vi "create_full_request_data.vi"(0 "llm_ollama_chatmodels in":refnum<class "llm_ollama_chatmodels.lvclass">, 5 "Messages":refnum<class "abstract_message_base.lvclass">[](array[class]), 11 "error in (no error)":errorcluster) -> (4 "llm_ollama_chatmodels out":refnum<class "llm_ollama_chatmodels.lvclass">, 6 "Request Data":string, 15 "error out":errorcluster)   [LabVIEW 2020, in "llm_ollama_chatmodels.lvclass"]
uses:
  llm_ollama_chatmodels.lvclass
  D:/Personal/LabVIEW LLMs/src/models/abstract_llm_base/abstract_llm_base.lvclass
  abstract_message_base/abstract_message_base.lvclass
  utils/ollama_chatmodel_request_data.ctl
  utils/ollama_options.ctl
  llm_ollama_chatmodels.lvclass/llm_ollama_chatmodels.ctl
  message_text/message_text.lvclass
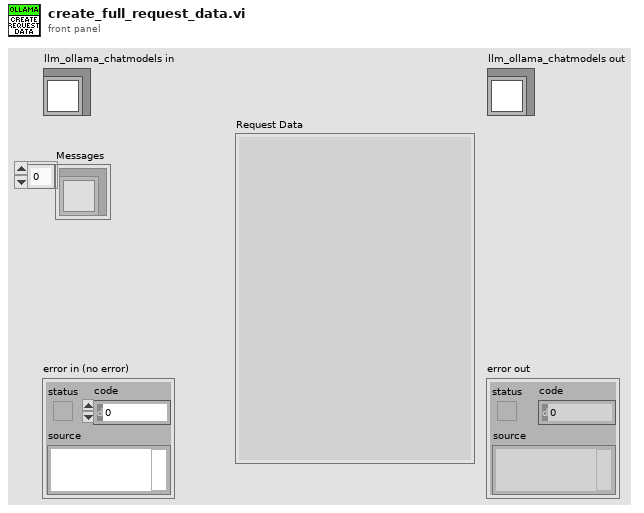
[diagram p1: front panel]
types:
  T1 = typedef "llm_ollama_chatmodels.lvclass/ollama_chatmodel_request_data.ctl" = cluster{"model":string, "messages":cluster{"role":string, "content":string}[], "stream":bool, "options":T2}
  T2 = typedef "llm_ollama_chatmodels.lvclass/ollama_options.ctl" = cluster{"temperature":dbl, "num_predict":i32, "top_p":dbl, "frequency_penalty":dbl, "presence_penalty":dbl, "seed":u32, "format":string}
  T3 = typedef "message_text.lvclass/message.ctl" = cluster{"role":string, "content":string[]}
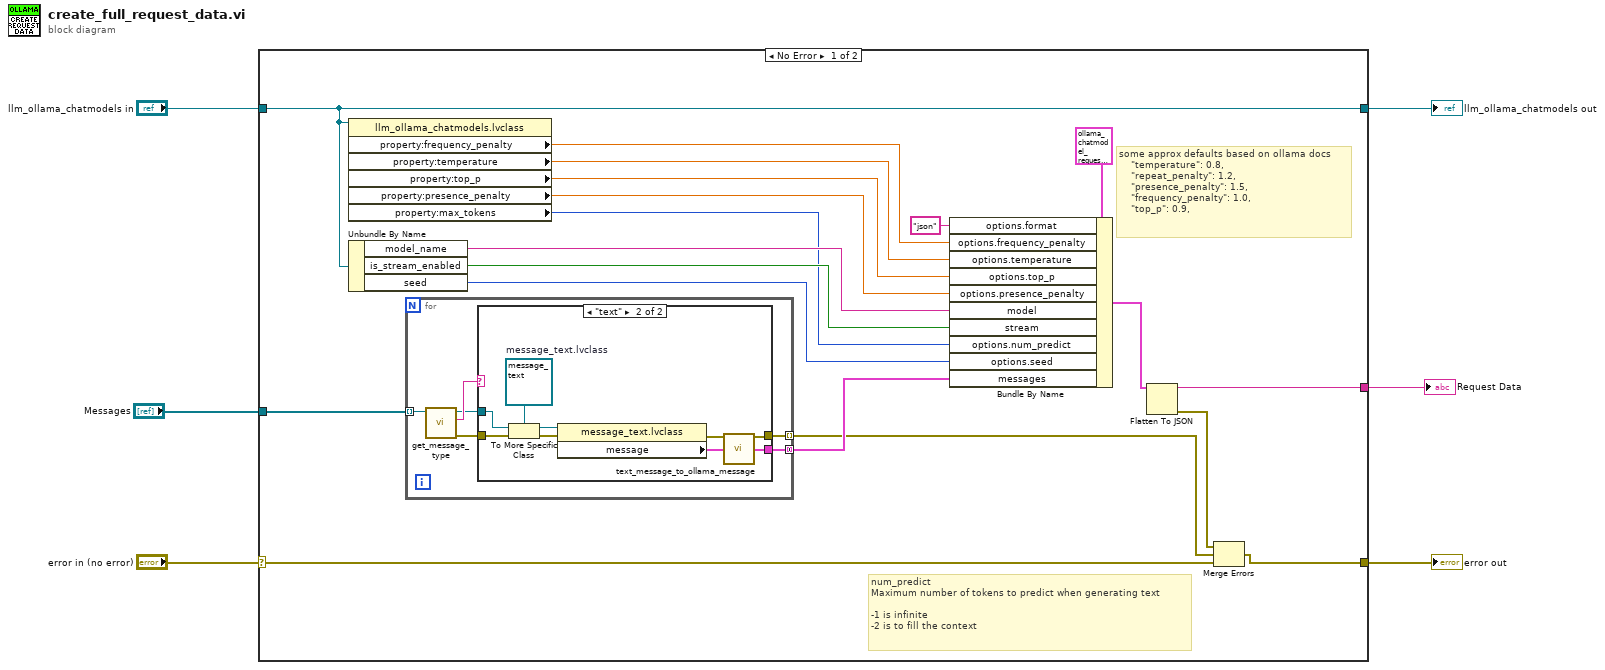
[diagram p0: block diagram]
diagram:
  n1 = case shown="No Error" "error in (no error)" {
    selector: "error in (no error)" -> [w25 w42]
    tunnel: [w20 w42] -> w5
    tunnel: [w13 w41] -> w3
    tunnel: "llm_ollama_chatmodels in" -> [w13 w41]
    tunnel: "Messages" -> [w23 _]
    tunnel: [w17 _] -> w1
    frame No Error {
      # "some approx defaults based on ollama docs\n    \"temperature\": 0.8,\n    \"repeat_penalty\": 1.2,\n    \"presence_penalty\": 1.5,\n    \"frequency_penalty\": 1.0,\n    \"top_p\": 0.9,"
      # "num_predict\nMaximum number of tokens to predict when generating text\n\n-1 is infinite\n-2 is to fill the context"
      n2 = property class="llm_ollama_chatmodels.lvclass"(reference=w13) -> ("property:frequency_penalty"=w12:dbl, "property:temperature"=w11:dbl, "property:top_p"=w10:dbl, "property:presence_penalty"=w9:dbl, "property:max_tokens"=w8:u32)  [unwired: 1 in, 2 out]
      n3 = Unbundle By Name(w13) -> ("model_name"=w16:string, "is_stream_enabled"=w15:bool, "seed"=w7:u32)
      n4 = for {
        tunnel: w23 -> [w31] mode=indexing
        tunnel: [w27] -> w19 mode=indexing
        tunnel: [w26] -> w22 mode=concatenating
        n5 = call-dynamic "get_message_type.vi"("abstract_message_base in"=w31) -> ("error out"=w28:errorcluster, "Type"=w30:string, "abstract_message_base out"=w29:refnum<class "abstract_message_base.lvclass">)  [unwired: 8 in]
        n6 = case shown="\"text\"" w30 {
          tunnel: w29 -> [_ w39]
          tunnel: w28 -> [w32 w40]
          tunnel: [w32 w35] -> w27
          tunnel: [_ w33] -> w26
          frame Default {
          }
          frame "text" {
            w38 = refnum<class "message_text.lvclass"> refnum  # message_text.lvclass
            n7 = To More Specific Class(target class=w38, reference=w39, error in=w40) -> (specific class reference=w37:refnum<class "message_text.lvclass">, error out=w36:errorcluster)
            n8 = property class="message_text.lvclass"(reference=w37, error in=w36) -> (error out=w35:errorcluster, "message"=w34:T3)  [unwired: 1 out]
            n9 = call "text_message_to_ollama_message.vi"("message"=w34) -> ("messages out"=w33:cluster{"role":string, "content":string}[])
          }
        }
      }
      n10 = Bundle By Name(cluster=T1 {"model"="", "messages"=[], "stream"=FALSE, "options"={"temperature"=1.0, "num_predict"=256, "top_p"=1.0, "frequency_penalty"=0.0, "presence_penalty"=0.0, "seed"=0, "format"="text"}} ("data"), "options.format"="json", "options.frequency_penalty"=w12, "options.temperature"=w11, "options.top_p"=w10, "options.presence_penalty"=w9, "model"=w16, "stream"=w15, "options.num_predict"=w8, "options.seed"=w7, "messages"=w22) -> (w21:T1)
      n11 = Flatten To JSON(anything=w21) -> (JSON string=w17:string, 11:w18:errorcluster)  [unwired: 2 in]
      n12 = Merge Errors(w18, w19, w25) -> (w20:errorcluster)
    }
    frame Error {
    }
  }
  "error out" <- w5
  "llm_ollama_chatmodels out" <- w3
  "Request Data" <- w1
